vi "change iterative coordinates.vi"() -> ()   [LabVIEW 2020]
uses:
  <vilib>/Analysis/NI_AALPro.lvlib
  <vilib>/Analysis/coordinate.llb/2D Cartesian Coordinate Rotation (Scalar).vi
panel:
  out "Array":dbl[][](array[numeric])
  in  "stop":bool
  in  "theta (degrees)":dbl
  in  "Rotate by angle":bool
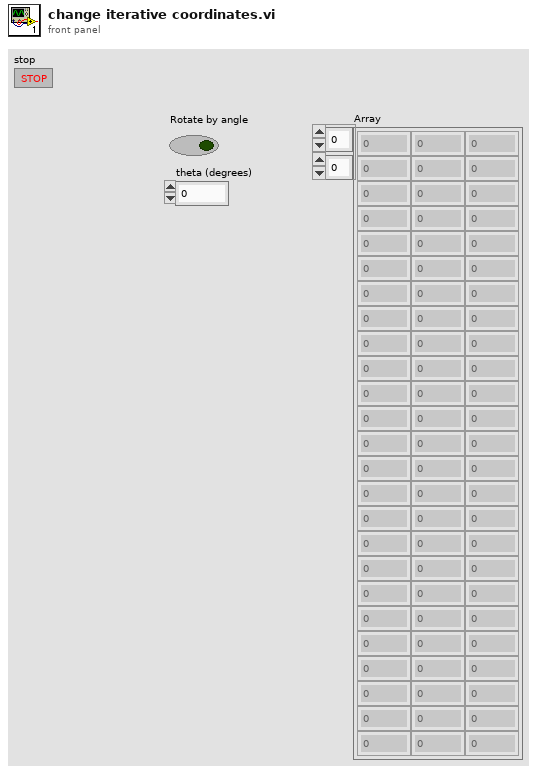
[diagram p1: front panel]
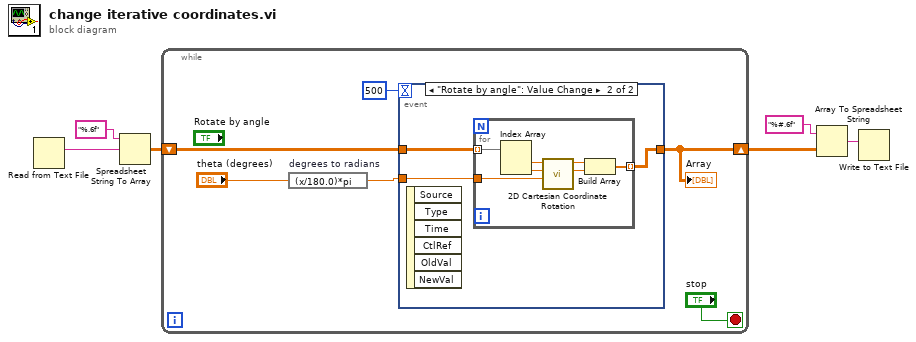
[diagram p0: block diagram]
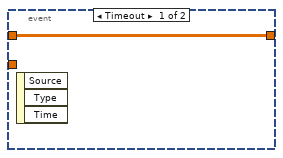
[diagram p2: hidden frame]
diagram:
  n1 = Read from Text File() -> (text=w6:string)  [unwired: 4 in, 3 out]
  n2 = Spreadsheet String To Array(format string="%.6f", spreadsheet string=w6) -> (array=w4:dbl[][])  [unwired: 2 in]
  n3 = while {
    shift-right: [w7] -> w1
    shift-left: w4 -> [w11]
    stop <- "stop" stop-if-true
    n4 = expression code="(x/180.0)*pi" "degrees to radians"("theta (degrees)") -> (w8:dbl)
    n5 = event shown="[1] \"Rotate by angle\": Value Change" {
      selector: _ -> [_ _]
      dyn-events: _ -> [_ _]
      timeout: 500 -> [_ _]
      tunnel: w11 -> [w13 w16]
      tunnel: [w13 w15] -> w7
      tunnel: w8 -> [_ w14]
      event Timeout {
        n6 = event-data() -> ()  [unwired: 1 in, 3 out]
      }
      event "Rotate by angle": Value Change {
        n7 = event-data() -> ()  [unwired: 1 in, 6 out]
        n8 = for {
          tunnel: w16 -> [w23] mode=indexing
          tunnel: [w22] -> w15 mode=indexing
          tunnel: w14 -> [w19]
          n9 = Index Array(array=w23) -> (element #1=w21:dbl, element #2=w20:dbl)  [unwired: 2 in]
          n10 = call-poly <vilib>:"2D Cartesian Coordinate Rotation.vi"("theta"=w19, "y"=w20, "x"=w21) -> ("y out"=w17:dbl, "x out"=w18:dbl)  [unwired: 6 in, 1 out]
          n11 = Build Array(w18, w17) -> (w22:dbl[])
        }
      }
    }
    "Array" <- w7
  }
  n12 = Array To Spreadsheet String(array=w1, 3:"%#.6f" ("format string")) -> (spreadsheet string=w3:string)  [unwired: 1 in]
  n13 = Write to Text File(text=w3) -> ()  [unwired: 3 in, 3 out]
